vi "Configure Burst.vi"(6 "Burst Phase (0.0 Degrees)":dbl, 7 "Enable Burst (F: Disable)":bool, 8 "error in (no error)":errorcluster, 9 "Burst Count (2)":i32=2, 10 "Channel (1: Channel1)":u16(ring)=1 items=["Channel1"=1, "Channel2"=2], 11 "VISA resource name":refnum<visa-resource-name>) -> (0 "error out":errorcluster, 3 "VISA resource name out":refnum<visa-resource-name>)   [LabVIEW 2009, in "Agilent 81150.lvlib"]
doc: "Allows and configures burst modulation. Configures the function generator to output a waveform with specified number of cycles, called burst. The carrier waveform shape and parameters are set by Configure Standard Waveform."
uses:
  Agilent 81150.lvlib
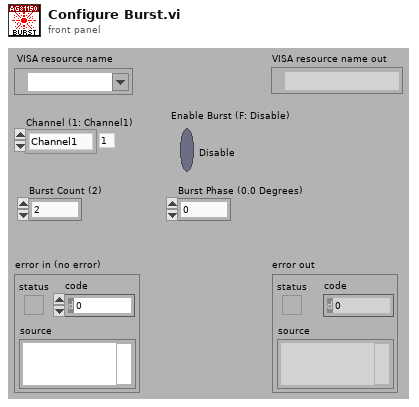
[diagram p1: front panel]
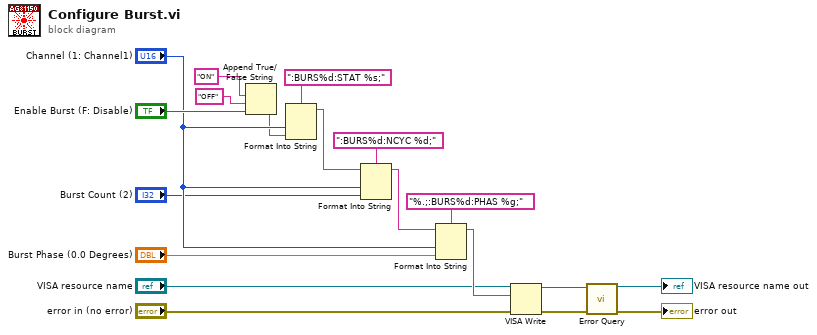
[diagram p0: block diagram]
diagram:
  n1 = Append True/False String(1:"Enable Burst (F: Disable)", 2:"OFF", 3:"ON") -> (0:w14:string)  [unwired: 1 out]
  n2 = Format Into String(format string=":BURS%d:STAT %s;", "Channel (1: Channel1)", w14) -> (resulting string=w12:string)  [unwired: 2 in, 1 out]
  n3 = Format Into String(format string=":BURS%d:NCYC %d;", initial string=w12, "Channel (1: Channel1)", "Burst Count (2)") -> (resulting string=w10:string)  [unwired: 1 in, 1 out]
  n4 = Format Into String(format string="%.;:BURS%d:PHAS %g;", initial string=w10, "Channel (1: Channel1)", "Burst Phase (0.0 Degrees)") -> (resulting string=w9:string)  [unwired: 1 in, 1 out]
  n5 = VISA Write(VISA resource name="VISA resource name", write buffer=w9, error in (no error)="error in (no error)") -> (VISA resource name out=w6:refnum<visa-resource-name>, error out=w5:errorcluster)  [unwired: 1 out]
  n6 = call "Error Query.vi"("error in (no error)"=w5, "VISA resource name"=w6) -> ("error out"=→"error out":errorcluster, "VISA resource name out"=→"VISA resource name out":refnum<visa-resource-name>)  [unwired: 8 out]
